vi "Robot_Simulation_Connect_Listen.vi"(8 "error in (no error)":errorcluster, 10 "timeout ms (25000)":i32, 11 "port":u16=3300) -> (0 "error out":errorcluster, 1 "Properties:Request URI":string, 2 "Properties:Return Headers":variant, 3 "WebSocket Connection out":refnum<class "websocket server.lvclass">)   [LabVIEW 2020]
uses:
  <vilib>/mediamongrels ltd/websockets/websockets/websocket server/websocket server.lvclass
  C:/Program Files (x86)/National Instruments/LabVIEW 2020/vi.lib/mediamongrels ltd/websockets/websockets/websocket/websocket.lvclass
  <vilib>/mediamongrels ltd/websockets/websockets/websocket/websocket.lvclass/websocket.ctl
  <vilib>/mediamongrels ltd/websockets/websockets/websocket server/websocket server.lvclass/websocket server.ctl
  <vilib>/mediamongrels ltd/websockets/websockets/websocket/read return headers.vi
  <vilib>/mediamongrels ltd/websockets/websockets/websocket server/read request uri.vi
  <vilib>/mediamongrels ltd/websockets/sockets/visa tcp listener/visa tcp listener.lvclass
  <vilib>/mediamongrels ltd/websockets/sockets/visa tcp socket/visa tcp.lvclass
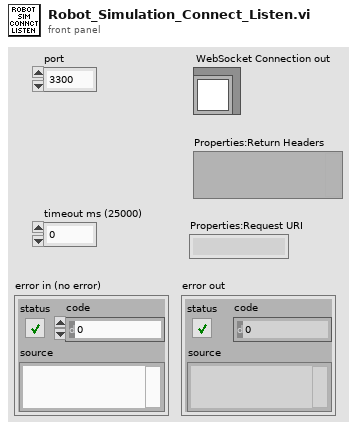
[diagram p1: front panel]
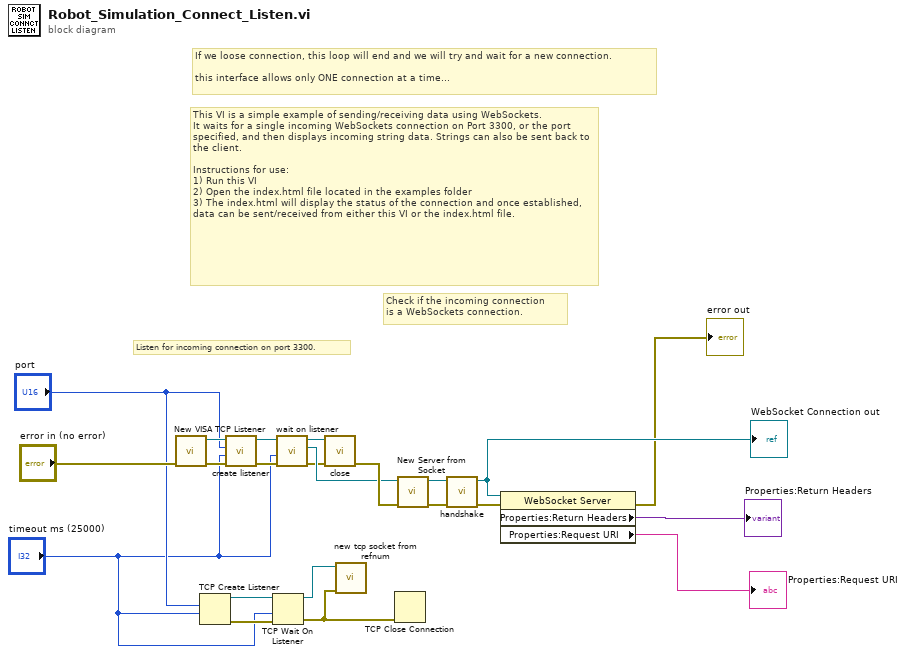
[diagram p0: block diagram]
diagram:
  # "If we loose connection, this loop will end and we will try and wait for a new connection.\n\nthis interface allows only ONE connection at a time..."
  # "This VI is a simple example of sending/receiving data using WebSockets.\nIt waits for a single incoming WebSockets connection on Port 3300, or the port specified, and then displays incoming string data. Strings can also be sent back to the client.\n\nInstructions for use:\n1) Run this VI\n2) Open the index.html file located in the examples folder\n3) The index.html will display the status of the connection and once established, data can be sent/received from either this VI or the index.html file."
  # "Check if the incoming connection\nis a WebSockets connection."
  # "Listen for incoming connection on port 3300."
  n1 = call <vilib>:"New VISA TCP Listener.vi"("error in (no error)"="error in (no error)") -> ("error out"=w15:errorcluster, "VISA TCP Listener out"=w14:refnum<class "visa tcp listener.lvclass">)  [unwired: 9 in]
  n2 = TCP Create Listener(9:"timeout ms (25000)", 10:"port") -> (0:w5:errorcluster, 3:w4:refnum<k5>)  [unwired: 3 in, 1 out]
  n3 = call-dynamic "create listener.vi"("error in (no error)"=w15, "timeout ms (5000)"="timeout ms (25000)", "Port"="port", "VISA TCP Listener in"=w14) -> ("error out"=w17:errorcluster, "VISA TCP Listener out"=w19:refnum<class "visa tcp listener.lvclass">)  [unwired: 6 in]
  n4 = TCP Wait On Listener(8:w5, 9:"timeout ms (25000)", 11:w4) -> (0:w1:errorcluster, 3:w2:refnum<k5>)  [unwired: 1 in, 3 out]
  n5 = call-dynamic "wait on listener.vi"("error in (no error)"=w17, "timeout ms (5000)"="timeout ms (25000)", "VISA TCP Listener in"=w19) -> ("error out"=w16:errorcluster, "Socket out"=w20:refnum<class "socket.lvclass">, "VISA TCP Listener out"=w18:refnum<class "visa tcp listener.lvclass">)  [unwired: 6 in]
  n6 = call-dynamic "close.vi"("error in (no error)"=w16, "VISA TCP Listener in"=w18) -> ("error out"=w21:errorcluster)  [unwired: 9 in]
  n7 = call <vilib>:"new tcp socket from refnum.vi"("error in (no error)"=w1, "TCP Network Connection Refnum"=w2) -> ()  [unwired: 8 in, 2 out]
  n8 = TCP Close Connection(error in (no error)=w1) -> ()  [unwired: 2 in, 2 out]
  n9 = call <vilib>:"New Server from Socket.vi"("error in (no error)"=w21, "Socket"=w20) -> ("error out"=w11:errorcluster, "WebSocket Server out"=w10:refnum<class "websocket server.lvclass">)  [unwired: 8 in]
  n10 = call-dynamic "handshake.vi"("error in (no error)"=w11, "WebSocket Connection in"=w10) -> ("error out"=w9:errorcluster, "WebSocket Connection out"=w22:refnum<class "websocket server.lvclass">)  [unwired: 8 in]
  "WebSocket Connection out" <- w22
  n11 = property class="WebSocket Server"(reference=w22, error in=w9) -> (error out=→"error out":errorcluster, "Properties:Return Headers"=→"Properties:Return Headers":variant, "Properties:Request URI"=→"Properties:Request URI":string)  [unwired: 1 out]
